vi "Create Known Hosts Collection Refnum.vi"(8 "error in (no error)":errorcluster, 11 "LIBSSH2_KNOWNHOSTS*":u64 format="%.0x") -> (0 "error out":errorcluster, 3 "known hosts collection":T1)   [LabVIEW 2013, in "libssh2.lvlib"]
uses:
  libssh2.lvlib
  Known Hosts Collection Refnum.ctl
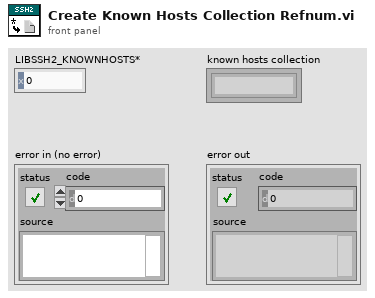
[diagram p1: front panel]
types:
  T1 = typedef "libssh2.lvlib/Known Hosts Collection Refnum.ctl" = refnum<k1>
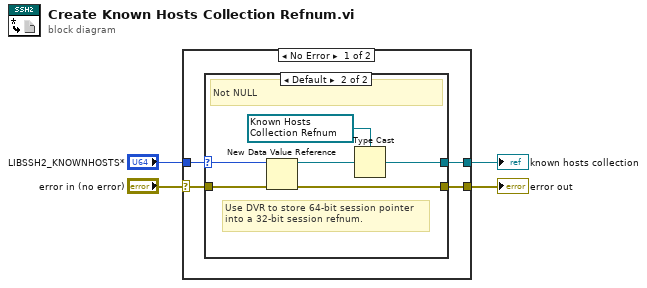
[diagram p0: block diagram]
diagram:
  n1 = case shown="No Error" "error in (no error)" {
    selector: "error in (no error)" -> [w6 w16]
    tunnel: [w8 _] -> w4
    tunnel: [w7 w16] -> w3
    tunnel: "LIBSSH2_KNOWNHOSTS*" -> [w5 _]
    frame No Error {
      n2 = case shown="Default" w5 {
        selector: w5 -> [_ w13]
        tunnel: [_ w14] -> w8
        tunnel: [w9 w11] -> w7
        tunnel: w6 -> [w9 w10]
        frame 0 {
          # "NULL"
        }
        frame Default {
          w15 = T1 refnum items=["Known Hosts"] ("known hosts collection")
          # "Use DVR to store 64-bit session pointer\ninto a 32-bit session refnum."
          # "Not NULL"
          n3 = New Data Value Reference(data value=w13, error in=w10) -> (data value reference=w12:refnum<data-value>, error out=w11:errorcluster)
          n4 = Type Cast(type=w15, x=w12) -> (*(type *) &x=w14:T1)
        }
      }
    }
    frame Error {
    }
  }
  "known hosts collection" <- w4
  "error out" <- w3
